vi "SetUSB5DoDataFifo.vi"(8 "错误输入（无错误）":errorcluster, 10 "Value":u32[](array[numeric]), 11 "DevIndex":i32) -> (0 "错误输出":errorcluster, 3 "DevIndex Out":i32)   [LabVIEW 2020]
uses:
  lib/x64/USB5000.dll
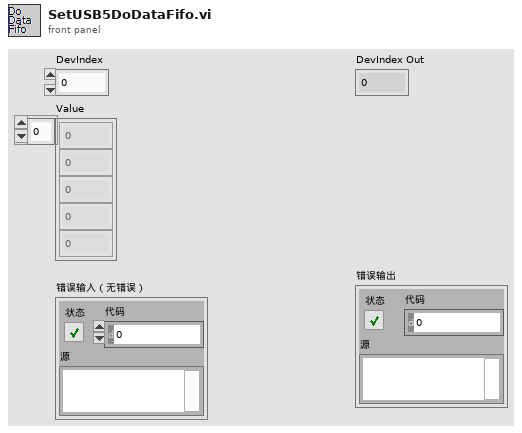
[diagram p1: front panel]
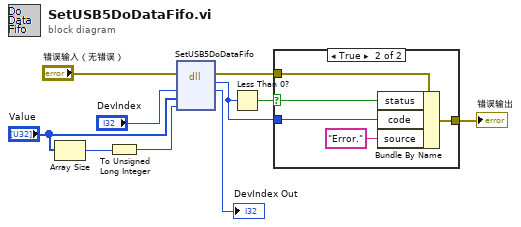
[diagram p0: block diagram]
diagram:
  n1 = Array Size(array="Value") -> (size(s)=w2:i32)
  n2 = To Unsigned Long Integer(number=w2) -> (unsigned 32bit integer=w1:u32)
  n3 = dll-call lib="C:/Users/phosense/Downloads/USB-5000/USB-5000_LabVIEW/lib/x64/USB5000.dll" fn="SetUSB5DoDataFifo"(error in="错误输入（无错误）", "DevIndex"="DevIndex", "Value"="Value", "Len"=w1) -> (error out=w6:errorcluster, "返回类型"=w5:i32, "DevIndex"=→"DevIndex Out":i32)  [unwired: 4 in, 1 out]
  n4 = Less Than 0?(x=w5) -> (x < 0?=w7:bool)
  n5 = case shown="True" w7 {
    selector: w7 -> [_ w12]
    tunnel: [w11 w14] -> w4
    tunnel: w5 -> [_ w16]
    tunnel: w6 -> [w11 w13]
    frame False {
    }
    frame True {
      n6 = Bundle By Name(cluster=w13, "status"=w12, "code"=w16, "source"="Error." ("error message (\"\")")) -> (w14:errorcluster)
    }
  }
  "错误输出" <- w4
